vi "Parse Empty Tag.vi"(8 "Error In":errorcluster) -> (0 "Error Out":errorcluster)   [LabVIEW 2018, in "Tests.lvlib" / "Lexer.lvlib"]
uses:
  Lexer.lvlib
  src/Toolkit/Low-Level/Tokens/EscapedVariable/EscapedVariable.lvclass
  src/Toolkit/Low-Level/Tokens/Keyable/API/Keyable.lvclass/Keyable.ctl
  src/Toolkit/Low-Level/Tokens/Keyable/API/Read Key.vi
  src/Toolkit/Low-Level/Support/Lex String.vi
  <vilib>/Utility/LVClass/Get LV Class Name.vi
  src/Toolkit/Low-Level/Tokens/Keyable/API/Keyable.lvclass
  <vilib>/addons/_JKI Toolkits/Caraya/classes/Test/Test.lvclass
  <vilib>/addons/_JKI Toolkits/Caraya/classes/Assert/Assert.lvclass
  Tests.lvlib
  src/Toolkit/Toolkit.lvlib
  src/Toolkit/Low-Level/Tokens/Abstract/Abstract.lvclass
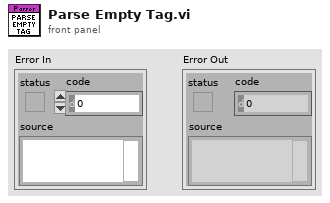
[diagram p1: front panel]
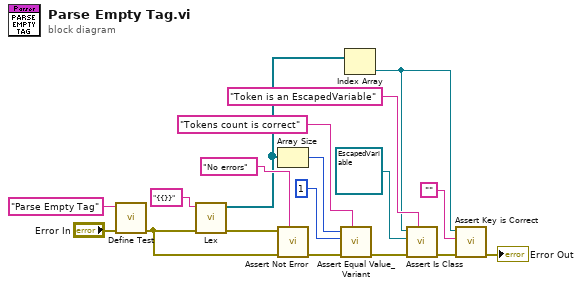
[diagram p0: block diagram]
diagram:
  n1 = call <vilib>:"Define Test.vi"("error in (no error)"="Error In", "Label (VI Title)"="Parse Empty Tag") -> ("error out"=w3:errorcluster)  [unwired: 9 in]
  n2 = call-poly "Lex.vi"("Error In"=w3, "Input"="{{}}") -> ("Error Out"=w16:errorcluster, "Tokens"=w1:refnum<class "Abstract.lvclass">[])  [unwired: 8 in]
  n3 = Array Size(array=w1) -> (size(s)=w12:i32)
  n4 = call <vilib>:"Assert Not Error.vi"("Label"="No errors", "error in (no error)"=w3, "Not Error?"=w16) -> ("error out"=w14:errorcluster)  [unwired: 8 in]
  n5 = call <vilib>:"Assert Equal Value_Variant.vi"("Label"="Tokens count is correct", "error in (no error)"=w14, "Y"=1 ("size(s)"), "X"=w12) -> ("error out"=w9:errorcluster)  [unwired: 7 in]
  n6 = Index Array(array=w1) -> (element=w4:refnum<class "Abstract.lvclass">)  [unwired: 1 in]
  n7 = call "Assert Is Class.vi"("Label"="Token is an EscapedVariable", "Error In"=w9, "Expected"=refnum<class "EscapedVariable.lvclass"> refnum ("Mustache.lvlib:Tokens.lvlib:Tag.lvclass"), "Actual"=w4) -> ("Error Out"=w5:errorcluster)  [unwired: 7 in]
  n8 = call "Assert Key is Correct.vi"("Error In"=w5, "Expected"="", "Token"=w4) -> ("Error Out"=→"Error Out":errorcluster)  [unwired: 8 in]
